vi "Top.vi"() -> ()   [LabVIEW 2013]
uses:
  <vilib>/Platform/TimedLoop/XDataNode/wakeup.ctl
  <vilib>/Platform/TimedLoop/XDataNode/XDNodeRunTimeDep.lvlib
  <vilib>/Platform/TimedLoop/XDataNode/nitl_modes.ctl
  <vilib>/Platform/TimedLoop/XDataNode/timing_clust.ctl
  <vilib>/Platform/TimedLoop/XDataNode/XDataNode.xnode
  <vilib>/eio/EIONode/EIONode.xnode
  <vilib>/rvi/eio/common/nirviEmuTemplateMethod_errors.vi
  <vilib>/NI/Engine Simulation Toolkit (EST)/APU/APU.lvlib
  <vilib>/NI/Engine Simulation Toolkit (EST)/ECU Event/Timing/ECU Event Timing.lvlib
  <vilib>/NI/Engine Simulation Toolkit (EST)/ECU Event/Timing/Capture Settings.ctl
  <vilib>/rvi/LocalResourceManager/LocalResourceManager.xnode
  <vilib>/rvi/eio/common/nirviEmuReportErrorAndStop.vi
  <vilib>/rvi/DataTransferAndStorage/Container/Common/niFpgaContainerGetUniqueNameForEmu.vi
  <vilib>/rvi/DataTransferAndStorage/Container/Common/niFpgaContainerSetEmuInfo.vi
  <vilib>/NI/Engine Simulation Toolkit (EST)/Digital Pattern Generation/Digital Pattern Generation.lvlib
  <vilib>/NI/Engine Simulation Toolkit (EST)/Digital Pattern Generation/Digital Pattern Generation.vi
  PWM/trunk/Source/IP/Typedefs/PWM.ctl
  <vilib>/NI/Engine Simulation Toolkit (EST)/APU/Settings.ctl
  <vilib>/NI/Engine Simulation Toolkit (EST)/APU/Input.ctl
  <vilib>/NI/Engine Simulation Toolkit (EST)/APU/Output.ctl
  <vilib>/NI/Engine Simulation Toolkit (EST)/APU/Shared Settings.ctl
  <vilib>/NI/Engine Simulation Toolkit (EST)/ECU Event/Timing/Capture Output.ctl
  <vilib>/NI/Engine Simulation Toolkit (EST)/ECU Event/Timing/Measure Settings.ctl
  <vilib>/NI/Engine Simulation Toolkit (EST)/ECU Event/Timing/Measure Output.ctl
  <vilib>/NI/Engine Simulation Toolkit (EST)/Digital Pattern Generation/Load Input.ctl
  <vilib>/NI/Engine Simulation Toolkit (EST)/Digital Pattern Generation/Input.ctl
  <vilib>/NI/Engine Simulation Toolkit (EST)/Digital Pattern Generation/Settings.ctl
panel:
  in  "settings.Cam Position":T1
  in  "input.Cam Position":T2
  in  "load input.Cam Position":T3
  in  "settings.Crank Position":T1
  in  "input.Crank Position":T2
  in  "load input.Crank Position":T3
  out "output.Fuel5.event 2":T4
  out "status.Fuel5":T5
  in  "settings.Fuel5":T6
  out "output.Fuel5.event 1":T4
  out "output.Fuel4.event 2":T4
  out "status.Fuel4":T5
  in  "settings.Fuel4":T6
  out "output.Fuel4.event 1":T4
  out "output.Fuel3.event 2":T4
  out "status.Fuel3":T5
  in  "settings.Fuel3":T6
  out "output.Fuel3.event 1":T4
  out "output.Fuel2.event 2":T4
  out "status.Fuel2":T5
  in  "settings.Fuel2":T6
  out "output.Fuel2.event 1":T4
  out "output.Fuel1.event 2":T4
  out "status.Fuel1":T5
  in  "settings.Fuel1":T6
  out "output.Fuel1.event 1":T4
  out "output.Fuel0.event 2":T4
  out "status.Fuel0":T5
  in  "settings.Fuel0":T6
  out "output.Fuel0.event 1":T4
  out "output.Spark6.event 2":T4
  out "status.Spark6":T5
  in  "settings.Spark6":T6
  out "output.Spark6.event 1":T4
  out "output.Spark5.event 2":T4
  out "status.Spark5":T5
  in  "settings.Spark5":T6
  out "output.Spark5.event 1":T4
  out "output.Spark4.event 2":T4
  out "status.Spark4":T5
  in  "settings.Spark4":T6
  out "output.Spark4.event 1":T4
  out "output.Spark3.event 2":T4
  out "status.Spark3":T5
  in  "settings.Spark3":T6
  out "output.Spark3.event 1":T4
  out "output.Spark2.event 2":T4
  out "status.Spark2":T5
  in  "settings.Spark2":T6
  out "output.Spark2.event 1":T4
  out "output.Spark1.event 2":T4
  out "status.Spark1":T5
  in  "settings.Spark1":T6
  out "output.Spark1.event 1":T4
  in  "shared settings.APU":T7 {"cycle start" format="%#.15g"}
  out "Output.APU":T8 caption="output"
  in  "Input.APU":T9 caption="input"
  in  "Settings.APU":T10
  in  "PWM write.Key Switch":T11
  in  "PWM write.Airflow":T11
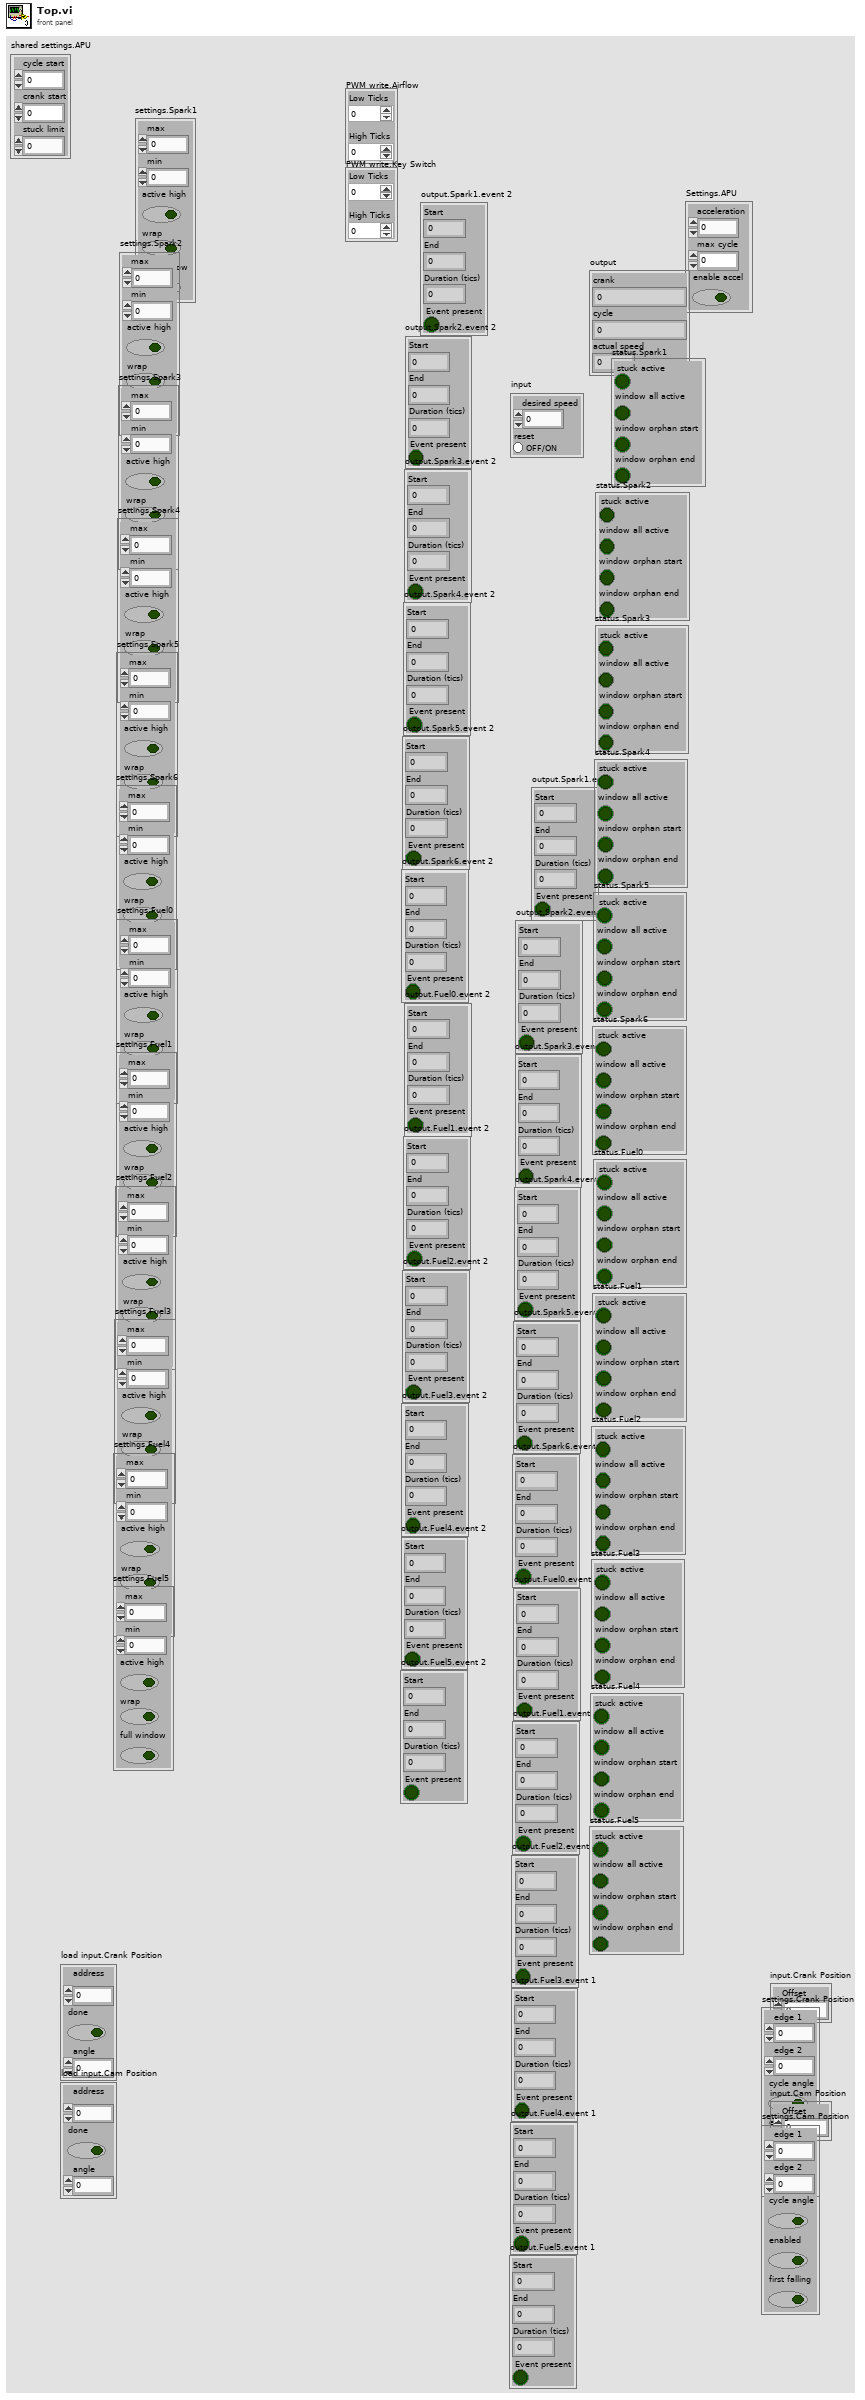
[diagram p1: front panel]
types:
  T1 = typedef "Engine Simulation Toolkit.lvlib/Digital Pattern Generation.lvlib/Settings.ctl" = cluster{"edge 1":u16, "edge 2":u16, "cycle angle":bool, "enabled":bool, "first falling":bool}
  T2 = typedef "Engine Simulation Toolkit.lvlib/Digital Pattern Generation.lvlib/Input.ctl" = cluster{"Offset":i16}
  T3 = typedef "Engine Simulation Toolkit.lvlib/Digital Pattern Generation.lvlib/Load Input.ctl" = cluster{"address":fxp<+,11,11>, "done":bool, "angle":u16}
  T4 = typedef "Engine Simulation Toolkit.lvlib/ECU Event Timing.lvlib/Capture Output.ctl" = cluster{"Start":u16, "End":u16, "Duration (tics)":fxp<+,18,18>, "Event present":bool}
  T5 = typedef "Engine Simulation Toolkit.lvlib/ECU Event Timing.lvlib/Measure Output.ctl" = cluster{"stuck active":bool, "window all active":bool, "window orphan start":bool, "window orphan end":bool}
  T6 = typedef "Engine Simulation Toolkit.lvlib/ECU Event Timing.lvlib/Measure Settings.ctl" = cluster{"max":u16, "min":u16, "active high":bool, "wrap":bool, "full window":bool}
  T7 = typedef "Engine Simulation Toolkit.lvlib/APU.lvlib/Shared Settings.ctl" = cluster{"cycle start":fxp<+,2,2>, "crank start":u16, "stuck limit":fxp<+,18,18>}
  T8 = typedef "Engine Simulation Toolkit.lvlib/APU.lvlib/Output.ctl" = cluster{"crank":u16, "cycle":u16, "actual speed":fxp<+/-,23,2>}
  T9 = typedef "Engine Simulation Toolkit.lvlib/APU.lvlib/Input.ctl" = cluster{"desired speed":fxp<+/-,23,2>, "reset":bool}
  T10 = typedef "Engine Simulation Toolkit.lvlib/APU.lvlib/Settings.ctl" = cluster{"acceleration":fxp<+,18,-20>, "max cycle":fxp<+,2,2>, "enable accel":bool}
  T11 = typedef "PWM.ctl" = cluster{"Low Ticks":u32, "High Ticks":u32}
  T12 = typedef "XDNodeRunTimeDep.lvlib/timing_clust.ctl" = cluster{"Expected End [f-1]":u64, "Actual End [f-1]":u64, "Finished Late? [f-1]":bool, "Expected End [i-1]":u64, "Actual End [i-1]":u64, "Finished Late? [i-1]":bool, "Expected Start [i]":u64, "Actual Start [i]":u64, "Expected Start [f]":u64, "Actual Start [f]":u64, "Source Name":string, "Structure Name":string, "Period":i64, "Deadline":i64, "Offset":i64, "Start":i64, "Priority":i32, "Timeout":i32, "Mode":T13, "Wakeup Reason":T14, "Error":errorcluster, "Source Type":string, "Secondary Source Type":string, "Global End Time":u64, "Global Start Time":u64, "Frame Duration":u64, "Iteration Duration":u64, "Assigned CPU":i32, "I/O Scan Engine Mode":u32}
  T13 = typedef "XDNodeRunTimeDep.lvlib/nitl_modes.ctl" = enum32{"No Change", "Process missed periods, maintain original phase", "Discard missed periods, maintain original phase", "Process missed periods, ignore original phase", "Discard missed periods, ignore original phase"}
  T14 = typedef "XDNodeRunTimeDep.lvlib/wakeup.ctl" = enum32{"Normal", "Aborted", "Asynchronous wakeup", "Timing source error", "Timed loop error", "Timeout"}
  T15 = typedef "Engine Simulation Toolkit.lvlib/Digital Pattern Generation.lvlib/Load Data.ctl" = cluster{"max address":fxp<+,11,11>, "memory":refnum<k21>}
  T16 = typedef "Engine Simulation Toolkit.lvlib/APU.lvlib/Register Bus.ctl" = cluster{"Speed":refnum<k21>, "Crank Angle":refnum<k21>, "Cycle Angle":refnum<k21>, "Crank Count":refnum<k21>, "Cycle Count":refnum<k21>, "1.25 MHz Counter":refnum<k21>, "shared settings":T7}
  T17 = typedef "Engine Simulation Toolkit.lvlib/ECU Event Timing.lvlib/Capture Settings.ctl" = u8
  T18 = typedef "Engine Simulation Toolkit.lvlib/ECU Event Timing.lvlib/Measured Data.ctl" = cluster{"start":u16, "end":u16, "duration (tics)":fxp<+,18,18>, "window end":bool, "window begin":bool, "pulse end":bool, "pulse #":u8}
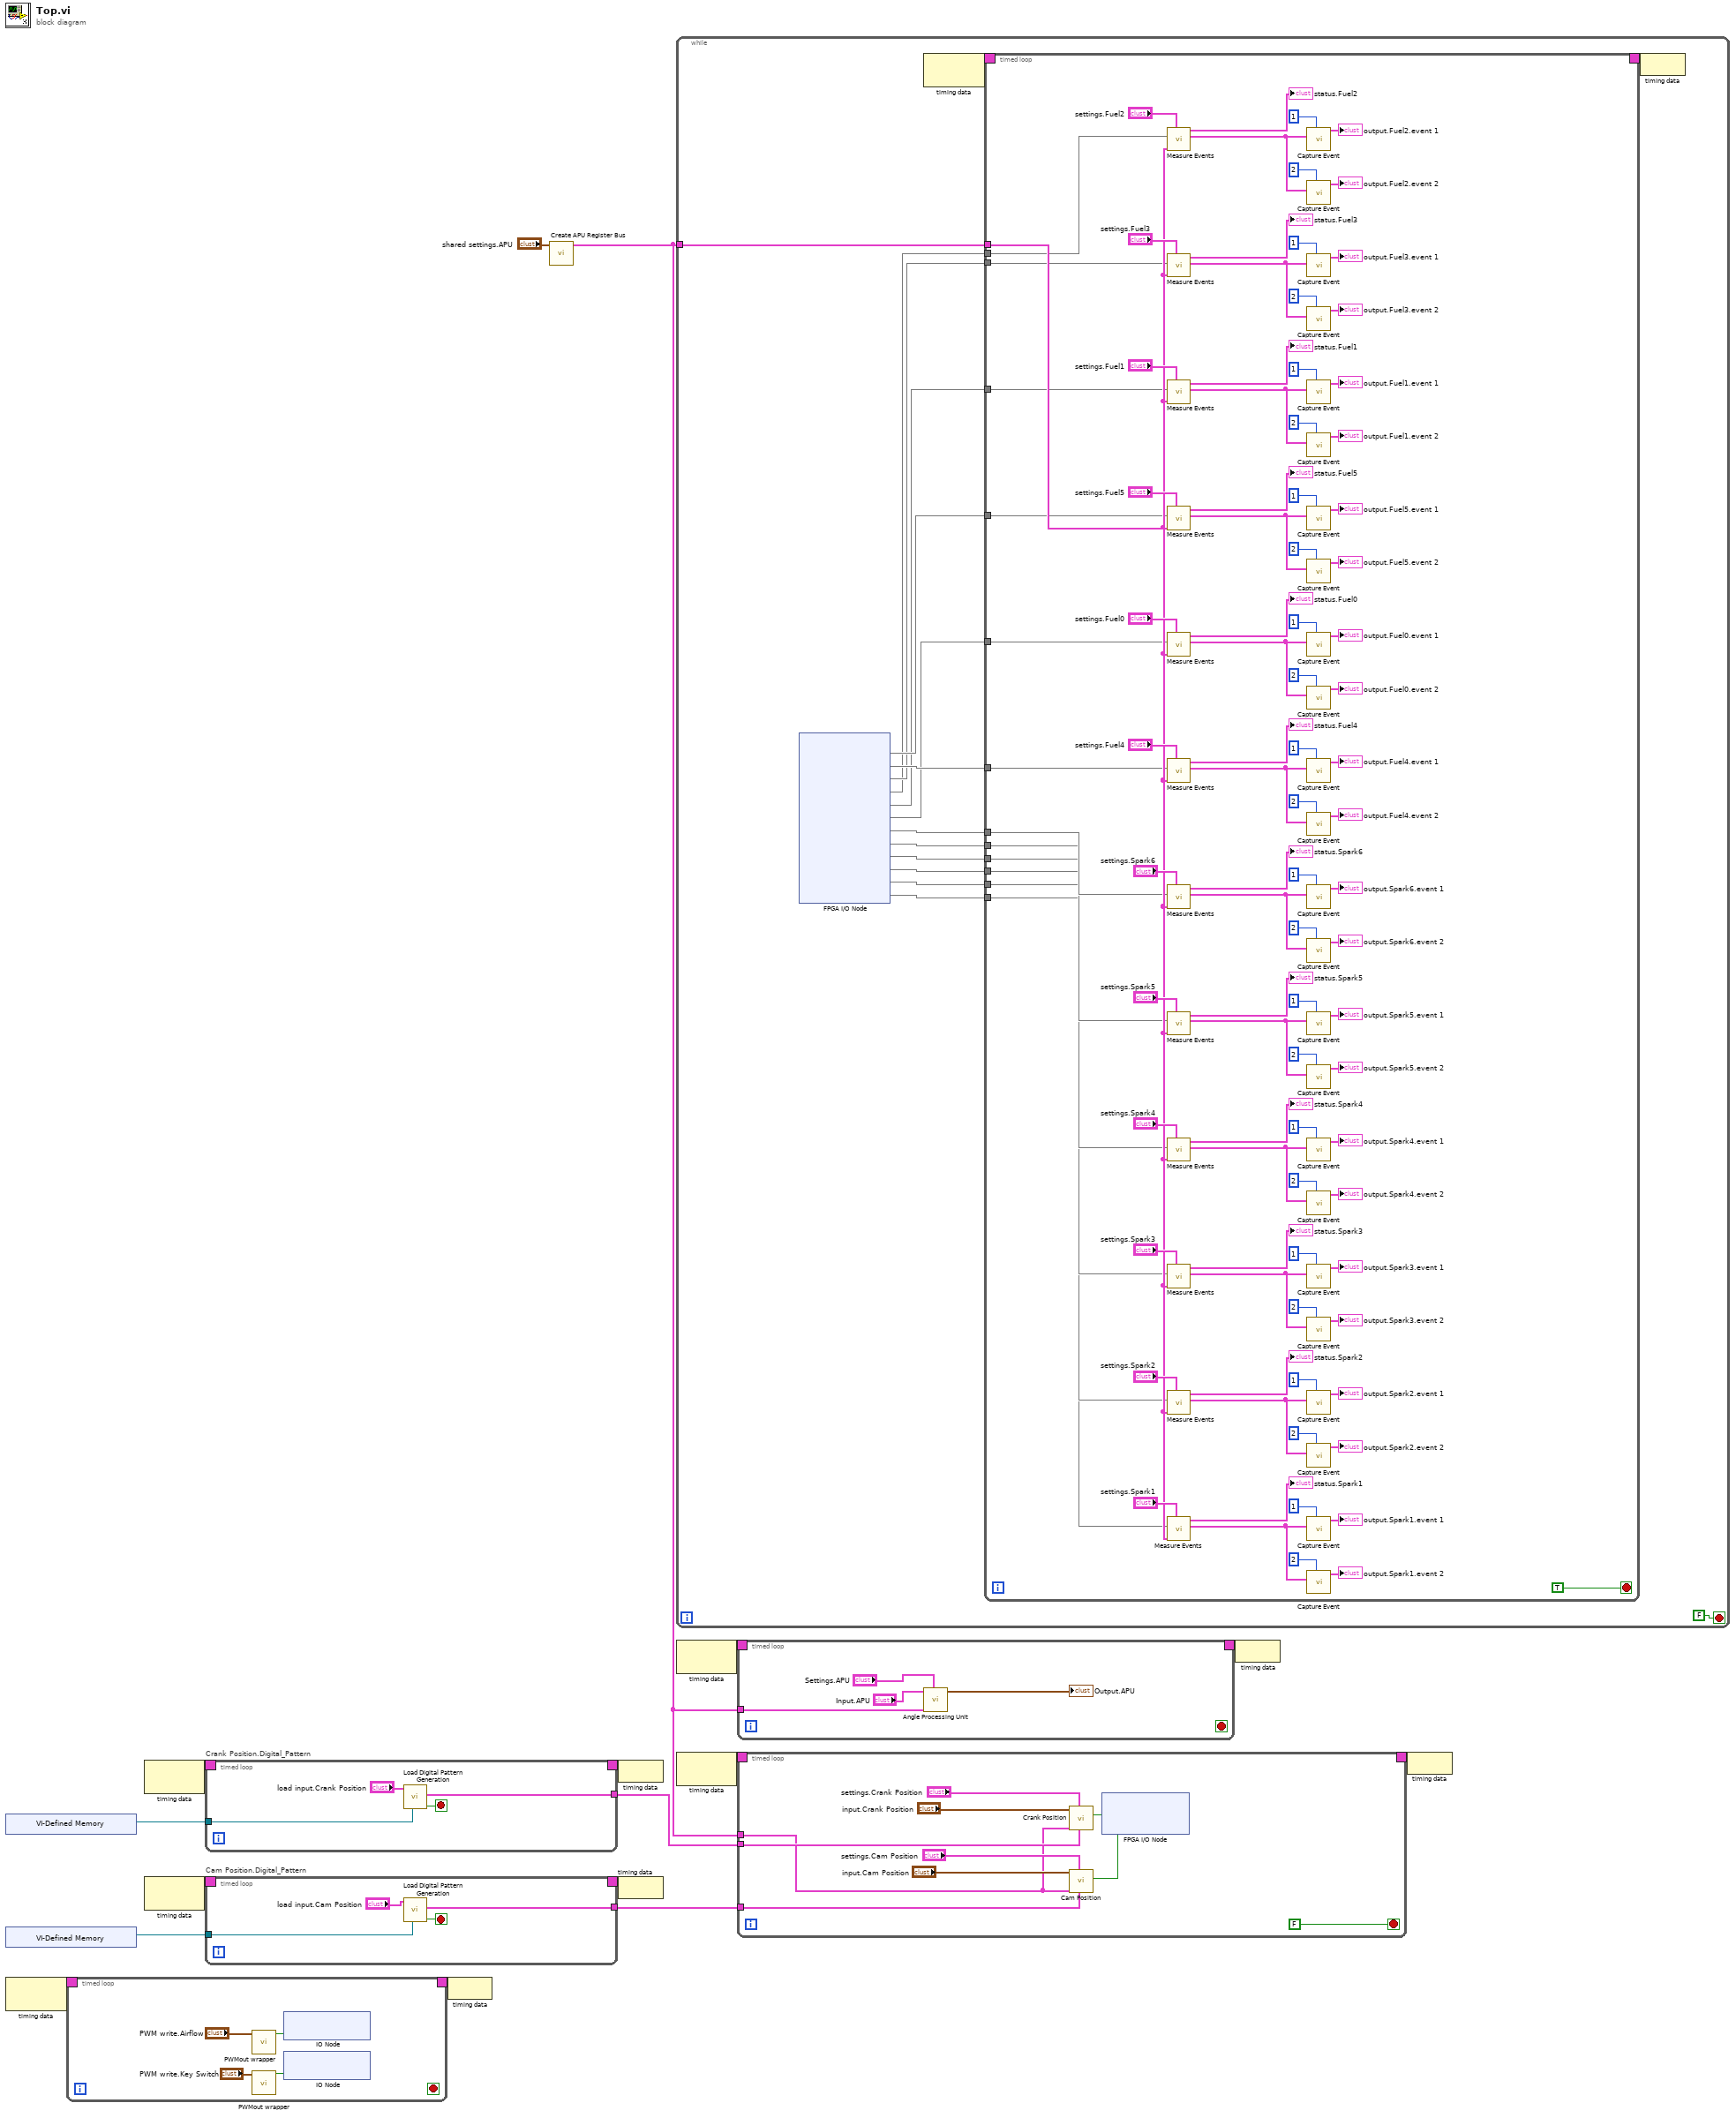
[diagram p0: block diagram]
diagram:
  n1 = xnode "VI-Defined Memory"() -> (w7:refnum<k21>)
  n2 = xnode "VI-Defined Memory"() -> (w4:refnum<k21>)
  n3 = node-c288() -> (w16:T12)  [unwired: 1 in]
  n4 = timed-loop "Timed Loop" {
    timing: w16 -> [_]
    timing-out: [_] -> w15
    stop <- _ stop-if-true
    n5 = call "PWMout wrapper.vi"(11:"PWM write.Airflow") -> (3:w20:bool)  [unwired: 10 in]
    n6 = call "PWMout wrapper.vi"(11:"PWM write.Key Switch") -> (3:w18:bool)  [unwired: 10 in]
    n7 = xnode ("IO Node")(w20) -> ()  [unwired: 1 in, 1 out]
    n8 = xnode ("IO Node")(w18) -> ()  [unwired: 1 in, 1 out]
  }
  n9 = node-c288() -> (w9:T12)  [unwired: 1 in]
  n10 = node-c288() -> (w6:T12)  [unwired: 1 in]
  n11 = timed-loop "Crank Position.Digital_Pattern" {
    timing: w9 -> [_]
    timing-out: [_] -> w8
    tunnel: w7 -> [w25]
    tunnel: [w24] -> w2
    stop <- w26 stop-if-true
    n12 = call <vilib>:"Load Digital Pattern Generation.vi"(6:w25, 11:"load input.Crank Position") -> (0:w26:bool, 2:w24:T15)  [unwired: 8 in]
  }
  n13 = timed-loop "Cam Position.Digital_Pattern" {
    timing: w6 -> [_]
    timing-out: [_] -> w5
    tunnel: w4 -> [w31]
    tunnel: [w30] -> w3
    stop <- w32 stop-if-true
    n14 = call <vilib>:"Load Digital Pattern Generation.vi"(6:w31, 11:"load input.Cam Position") -> (0:w32:bool, 2:w30:T15)  [unwired: 8 in]
  }
  n15 = node-c288(w15) -> ()
  n16 = call <vilib>:"Create APU Register Bus.vi"(11:"shared settings.APU") -> (3:w1:T16)  [unwired: 10 in]
  n17 = node-c288(w8) -> ()
  n18 = node-c288(w5) -> ()
  n19 = while "NI 9403" {
    tunnel: w1 -> [w47]
    stop <- FALSE stop-if-true
    n20 = xnode "FPGA I/O Node"() -> (w46, w45, w44, w43, w42, w41, w40, w39, w38, w37, w36, w35)  [unwired: 12 in, 12 out]
    n21 = node-c288() -> (w49:T12)  [unwired: 1 in]
    n22 = timed-loop "9403" {
      timing: w49 -> [_]
      timing-out: [_] -> w48
      tunnel: w47 -> [w63]
      tunnel: w46 -> [w62]
      tunnel: w45 -> [w61]
      tunnel: w44 -> [w60]
      tunnel: w43 -> [w59]
      tunnel: w42 -> [w58]
      tunnel: w41 -> [w57]
      tunnel: w40 -> [w56]
      tunnel: w39 -> [w55]
      tunnel: w38 -> [w54]
      tunnel: w37 -> [w53]
      tunnel: w36 -> [w52]
      tunnel: w35 -> [w51]
      stop <- TRUE stop-if-true
      n23 = call <vilib>:"Measure Events.vi"(7:"settings.Fuel2", 8:w63, 10:w59) -> (2:w88:T18, 3:→"status.Fuel2":T5)  [unwired: 7 in]
      n24 = call <vilib>:"Measure Events.vi"(7:"settings.Fuel3", 8:w63, 10:w60) -> (2:w81:T18, 3:→"status.Fuel3":T5)  [unwired: 7 in]
      n25 = call <vilib>:"Measure Events.vi"(7:"settings.Fuel1", 8:w63, 10:w58) -> (2:w95:T18, 3:→"status.Fuel1":T5)  [unwired: 7 in]
      n26 = call <vilib>:"Measure Events.vi"(7:"settings.Fuel5", 8:w63, 10:w62) -> (2:w67:T18, 3:→"status.Fuel5":T5)  [unwired: 7 in]
      n27 = call <vilib>:"Measure Events.vi"(7:"settings.Fuel0", 8:w63, 10:w57) -> (2:w102:T18, 3:→"status.Fuel0":T5)  [unwired: 7 in]
      n28 = call <vilib>:"Measure Events.vi"(7:"settings.Fuel4", 8:w63, 10:w61) -> (2:w74:T18, 3:→"status.Fuel4":T5)  [unwired: 7 in]
      n29 = call <vilib>:"Measure Events.vi"(7:"settings.Spark6", 8:w63, 10:w56) -> (2:w109:T18, 3:→"status.Spark6":T5)  [unwired: 7 in]
      n30 = call <vilib>:"Measure Events.vi"(7:"settings.Spark5", 8:w63, 10:w55) -> (2:w116:T18, 3:→"status.Spark5":T5)  [unwired: 7 in]
      n31 = call <vilib>:"Measure Events.vi"(7:"settings.Spark4", 8:w63, 10:w54) -> (2:w123:T18, 3:→"status.Spark4":T5)  [unwired: 7 in]
      n32 = call <vilib>:"Measure Events.vi"(7:"settings.Spark3", 8:w63, 10:w53) -> (2:w130:T18, 3:→"status.Spark3":T5)  [unwired: 7 in]
      n33 = call <vilib>:"Measure Events.vi"(7:"settings.Spark2", 8:w63, 10:w52) -> (2:w137:T18, 3:→"status.Spark2":T5)  [unwired: 7 in]
      n34 = call <vilib>:"Measure Events.vi"(7:"settings.Spark1", 8:w63, 10:w51) -> (2:w144:T18, 3:→"status.Spark1":T5)  [unwired: 7 in]
      n35 = call <vilib>:"Capture Event.vi"(7:T17 1 ("Settings.spark 1 shot 1"), 10:w88) -> (3:→"output.Fuel2.event 1":T4)  [unwired: 9 in]
      n36 = call <vilib>:"Capture Event.vi"(7:T17 2 ("name"), 10:w88) -> (3:→"output.Fuel2.event 2":T4)  [unwired: 9 in]
      n37 = call <vilib>:"Capture Event.vi"(7:T17 1 ("Settings.spark 1 shot 1"), 10:w81) -> (3:→"output.Fuel3.event 1":T4)  [unwired: 9 in]
      n38 = call <vilib>:"Capture Event.vi"(7:T17 2 ("name"), 10:w81) -> (3:→"output.Fuel3.event 2":T4)  [unwired: 9 in]
      n39 = call <vilib>:"Capture Event.vi"(7:T17 1 ("Settings.spark 1 shot 1"), 10:w95) -> (3:→"output.Fuel1.event 1":T4)  [unwired: 9 in]
      n40 = call <vilib>:"Capture Event.vi"(7:T17 2 ("name"), 10:w95) -> (3:→"output.Fuel1.event 2":T4)  [unwired: 9 in]
      n41 = call <vilib>:"Capture Event.vi"(7:T17 1 ("Settings.spark 1 shot 1"), 10:w67) -> (3:→"output.Fuel5.event 1":T4)  [unwired: 9 in]
      n42 = call <vilib>:"Capture Event.vi"(7:T17 2 ("name"), 10:w67) -> (3:→"output.Fuel5.event 2":T4)  [unwired: 9 in]
      n43 = call <vilib>:"Capture Event.vi"(7:T17 1 ("Settings.spark 1 shot 1"), 10:w102) -> (3:→"output.Fuel0.event 1":T4)  [unwired: 9 in]
      n44 = call <vilib>:"Capture Event.vi"(7:T17 2 ("name"), 10:w102) -> (3:→"output.Fuel0.event 2":T4)  [unwired: 9 in]
      n45 = call <vilib>:"Capture Event.vi"(7:T17 1 ("Settings.spark 1 shot 1"), 10:w74) -> (3:→"output.Fuel4.event 1":T4)  [unwired: 9 in]
      n46 = call <vilib>:"Capture Event.vi"(7:T17 2 ("name"), 10:w74) -> (3:→"output.Fuel4.event 2":T4)  [unwired: 9 in]
      n47 = call <vilib>:"Capture Event.vi"(7:T17 1 ("Settings.spark 1 shot 1"), 10:w109) -> (3:→"output.Spark6.event 1":T4)  [unwired: 9 in]
      n48 = call <vilib>:"Capture Event.vi"(7:T17 2 ("name"), 10:w109) -> (3:→"output.Spark6.event 2":T4)  [unwired: 9 in]
      n49 = call <vilib>:"Capture Event.vi"(7:T17 1 ("Settings.spark 1 shot 1"), 10:w116) -> (3:→"output.Spark5.event 1":T4)  [unwired: 9 in]
      n50 = call <vilib>:"Capture Event.vi"(7:T17 2 ("name"), 10:w116) -> (3:→"output.Spark5.event 2":T4)  [unwired: 9 in]
      n51 = call <vilib>:"Capture Event.vi"(7:T17 1 ("Settings.spark 1 shot 1"), 10:w123) -> (3:→"output.Spark4.event 1":T4)  [unwired: 9 in]
      n52 = call <vilib>:"Capture Event.vi"(7:T17 2 ("name"), 10:w123) -> (3:→"output.Spark4.event 2":T4)  [unwired: 9 in]
      n53 = call <vilib>:"Capture Event.vi"(7:T17 1 ("Settings.spark 1 shot 1"), 10:w130) -> (3:→"output.Spark3.event 1":T4)  [unwired: 9 in]
      n54 = call <vilib>:"Capture Event.vi"(7:T17 2 ("name"), 10:w130) -> (3:→"output.Spark3.event 2":T4)  [unwired: 9 in]
      n55 = call <vilib>:"Capture Event.vi"(7:T17 1 ("Settings.spark 1 shot 1"), 10:w137) -> (3:→"output.Spark2.event 1":T4)  [unwired: 9 in]
      n56 = call <vilib>:"Capture Event.vi"(7:T17 2 ("name"), 10:w137) -> (3:→"output.Spark2.event 2":T4)  [unwired: 9 in]
      n57 = call <vilib>:"Capture Event.vi"(7:T17 1 ("Settings.spark 1 shot 1"), 10:w144) -> (3:→"output.Spark1.event 1":T4)  [unwired: 9 in]
      n58 = call <vilib>:"Capture Event.vi"(7:T17 2 ("name"), 10:w144) -> (3:→"output.Spark1.event 2":T4)  [unwired: 9 in]
    }
    n59 = node-c288(w48) -> ()
  }
  n60 = node-c288() -> (w14:T12)  [unwired: 1 in]
  n61 = node-c288() -> (w11:T12)  [unwired: 1 in]
  n62 = timed-loop "Timed Loop" {
    timing: w14 -> [_]
    timing-out: [_] -> w13
    tunnel: w1 -> [w154]
    stop <- _ stop-if-true
    n63 = call <vilib>:"Angle Processing Unit.vi"(7:"Settings.APU", 8:w154, 11:"Input.APU") -> (3:→"Output.APU":T8)  [unwired: 8 in]
  }
  n64 = timed-loop "Timed Loop" {
    timing: w11 -> [_]
    timing-out: [_] -> w10
    tunnel: w3 -> [w161]
    tunnel: w2 -> [w160]
    tunnel: w1 -> [w159]
    stop <- FALSE stop-if-true
    n65 = call "Crank Position"(6:w160, 7:"settings.Crank Position", 8:w159, 11:"input.Crank Position") -> (2:w165:bool)  [unwired: 7 in]
    n66 = call "Cam Position"(6:w161, 7:"settings.Cam Position", 8:w159, 11:"input.Cam Position") -> (2:w162:bool)  [unwired: 7 in]
    n67 = xnode ("FPGA I/O Node")(w165, w162) -> ()  [unwired: 2 in, 2 out]
  }
  n68 = node-c288(w13) -> ()
  n69 = node-c288(w10) -> ()
